vi "fgv_timer_buff.vi"(7 "cmd":enum16{"write", "read"}(ring), 11 "time_status in":T1 {"total time" format="%.1f"; "run time" format="%.1f"; "wait time" format="%.1f"}) -> (3 "time_status out":T1 {"total time" format="%.1f"; "run time" format="%.1f"; "wait time" format="%.1f"})   [LabVIEW 2019]
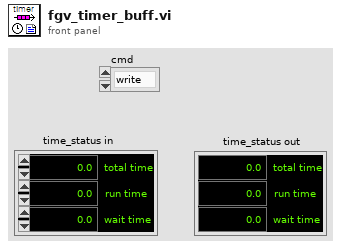
[diagram p1: front panel]
types:
  T1 = cluster{"total time":dbl, "run time":dbl, "wait time":dbl}
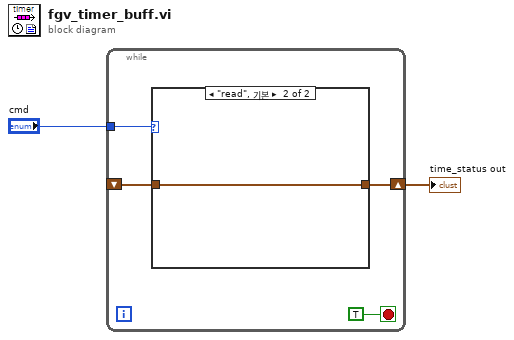
[diagram p0: block diagram]
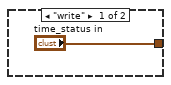
[diagram p2: hidden frame]
diagram:
  n1 = while {
    tunnel: "cmd" -> [w5]
    shift-right: [w4] -> w1
    shift-left: _ -> [w3]
    stop <- TRUE stop-if-true
    n2 = case shown="\"read\", 기본" w5 {
      tunnel: ["time_status in" w8] -> w4
      tunnel: w3 -> [_ w8]
      frame "write" {
      }
      frame "read", Default {
      }
    }
  }
  "time_status out" <- w1
